vi "PQinitSSL.vi"(8 "error in (no error)":errorcluster, 11 "do_init":i32) -> (0 "error out":errorcluster)   [LabVIEW 2019, in "libpqlv64.lvlib"]
uses:
  libpqlv64.lvlib
  libpq.dll
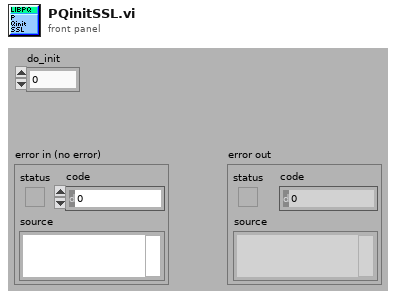
[diagram p1: front panel]
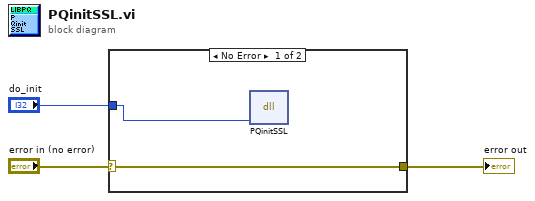
[diagram p0: block diagram]
diagram:
  n1 = case shown="No Error" "error in (no error)" {
    selector: "error in (no error)" -> [w5 w6]
    tunnel: [w5 w6] -> w2
    tunnel: "do_init" -> [w4 _]
    frame No Error {
      n2 = dll-call lib="libpq.*" fn="PQinitSSL"("do_init"=w4) -> ()  [unwired: 5 in, 2 out]
    }
    frame Error {
    }
  }
  "error out" <- w2
